vi "Normalize2DGaussianParameters.vi"(1 "best fit parameters IN":dbl[](array[numeric])) -> (0 "best fit parameters OUT":dbl[](array[numeric]))   [LabVIEW 2015]
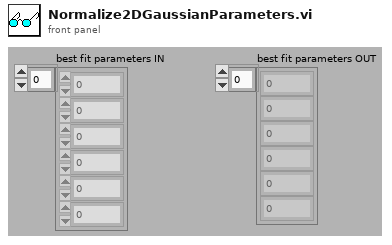
[diagram p1: front panel]
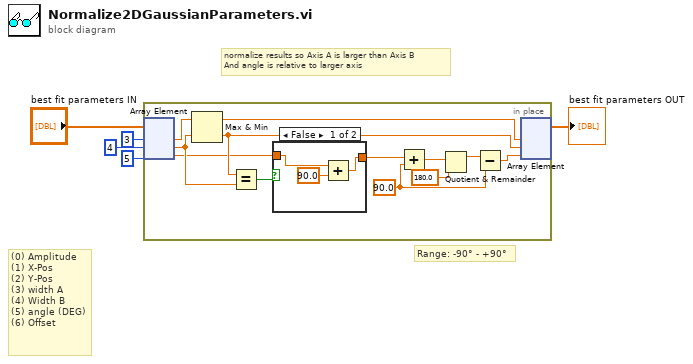
[diagram p0: block diagram]
diagram:
  # "(0) Amplitude\n(1) X-Pos\n(2) Y-Pos\n(3) width A\n(4) Width B\n(5) angle (DEG)\n(6) Offset"
  # "Range: -90° - +90°"
  # "normalize results so Axis A is larger than Axis B\nAnd angle is relative to larger axis"
  n1 = in-place {
    w11 = 90.0 ("y")
    n2 = in-place-array #1("best fit parameters IN", 3, 4, 5) -> (w17:dbl, w9:dbl, w7:dbl)
    n3 = Max & Min(x=w17, y=w9) -> (max(x,y)=w16:dbl, min(x,y)=w10:dbl)
    n4 = Equal?(x=w10, y=w9) -> (x = y?=w8:bool)
    n5 = case shown="False" w8 {
      tunnel: w7 -> [w19 w21]
      tunnel: [w20 w21] -> w6
      frame False {
        n6 = Add(x=w19, y=90.0) -> (x+y=w20:dbl)
      }
      frame True {
      }
    }
    n7 = Add(x=w6, y=w11) -> (x+y=w14:dbl)
    n8 = Quotient & Remainder(x=w14, y=180.0) -> (x-y*floor(x/y)=w13:dbl)  [unwired: 1 out]
    n9 = Subtract(x=w13, y=w11) -> (x-y=w12:dbl)
    n10 = in-place-array #1(w16, w10, w12) -> (→"best fit parameters OUT":dbl[])  [unwired: 3 out]
  }
